vi "To Message Name.vi"(3 "well known type":T1) -> (0 "message url":string, 1 "message name":string)   [LabVIEW 2019, in "grpc-lvsupport.lvlib"]
uses:
  grpc-lvsupport.lvlib
  Well Known Types.ctl
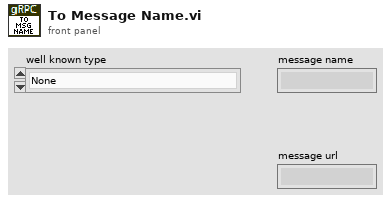
[diagram p1: front panel]
types:
  T1 = typedef "grpc-lvsupport.lvlib/Well Known Types.ctl" = enum32{"None", "Double2DArray", "String2DArray"}
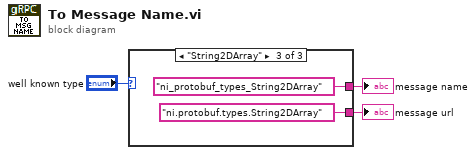
[diagram p0: block diagram]
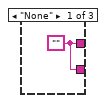
[diagram p2: hidden frame]
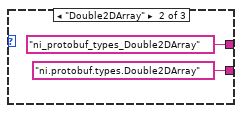
[diagram p3: hidden frame]
diagram:
  n1 = case shown="\"String2DArray\"" "well known type" {
    tunnel: [w4 "ni_protobuf_types_Double2DArray" ("message name") "ni_protobuf_types_String2DArray" ("message name")] -> w2
    tunnel: [w4 "ni.protobuf.types.Double2DArray" ("message name") "ni.protobuf.types.String2DArray" ("message name")] -> w1
    frame "None" {
      w4 = ""
    }
    frame "Double2DArray" {
    }
    frame "String2DArray" {
    }
  }
  "message name" <- w2
  "message url" <- w1
